vi "VoltScaleInfo.vi"(0 "refnum":refnum<file>, 11 "offset":i32) -> (2 "Votage scaling":T1, 4 "dup refnum":refnum<file>, 6 "Digitizer (dB)":sgl, 8 "Gain (dB)":sgl, 10 "Atten (dB)":sgl)   [LabVIEW 2022 SP3]
panel:
  out "blank":string
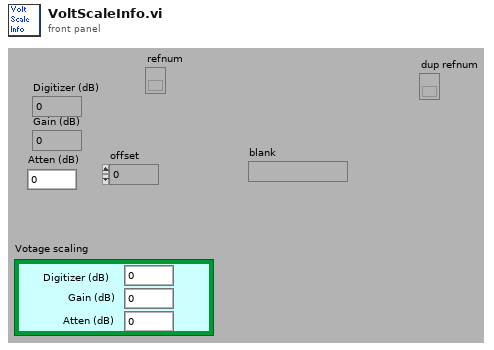
[diagram p1: front panel]
types:
  T1 = cluster{"Digitizer (dB)":sgl, "Gain (dB)":sgl, "Atten (dB)":sgl}
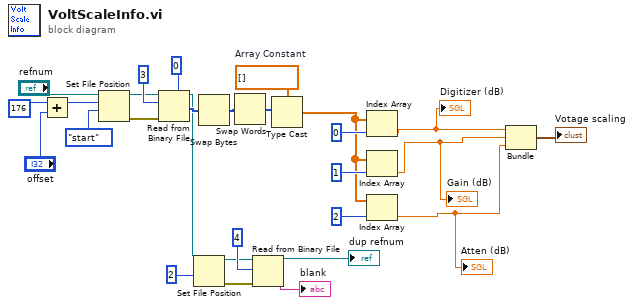
[diagram p0: block diagram]
diagram:
  w11 = sgl[] []  # Array Constant
  n1 = Add(x=176 ("pos offset (0)"), y="offset") -> (x+y=w20:i32)
  n2 = Set File Position(offset (in bytes) (0)=w20, refnum="refnum", from (0:start)=enum16{"start", "end", "current"}."start" ("pos mode (0:2)")) -> (refnum out=w17:refnum<file>, error out=w16:errorcluster)  [unwired: 1 in]
  n3 = Read from Binary File(5:0 ("byte stream type"), 8:w16, 10:3 ("count"), 11:w17) -> (2:w7:i32[], 3:w6:refnum<file>)  [unwired: 4 out]
  n4 = Set File Position(refnum=w6, from (0:start)=2) -> (refnum out=w19:refnum<file>, error out=w18:errorcluster)  [unwired: 1 in, 1 out]
  n5 = Swap Bytes(anything=w7) -> (byte swapped=w12:i32[])
  n6 = Swap Words(1:w12) -> (0:w10:i32[])
  n7 = Read from Binary File(8:w18, 10:4 ("count"), 11:w19) -> (2:→"blank":string, 3:→"dup refnum":refnum<file>)  [unwired: 5 out]
  n8 = Type Cast(type=w11, x=w10) -> (*(type *) &x=w4:sgl[])
  n9 = Index Array(array=w4, index=0) -> (element=w9:sgl)
  "Digitizer (dB)" <- w9
  n10 = Index Array(array=w4, index=1) -> (element=w8:sgl)
  "Gain (dB)" <- w8
  n11 = Index Array(array=w4, index=2) -> (element=w3:sgl)
  "Atten (dB)" <- w3
  n12 = Bundle(w9, w8, w3) -> (→"Votage scaling":cluster{sgl, sgl, sgl})  [unwired: 1 out]
